vi "Base Run Java Script.vi"(4 "error in":errorcluster, 5 "script args in":string, 6 "script name in":string, 7 "ATS Framework Fields in":T2) -> (0 "error out":errorcluster, 2 "run tool out":T1, 3 "ATS Framework Fields out":T2)   [LabVIEW 2019]
uses:
  <vilib>/Arcadia/Common/Framework/ATS Framework Fields.ctl
  <vilib>/Arcadia/Common/Framework/Run Tool Output.ctl
  <vilib>/Utility/error.llb/whitespace.ctl
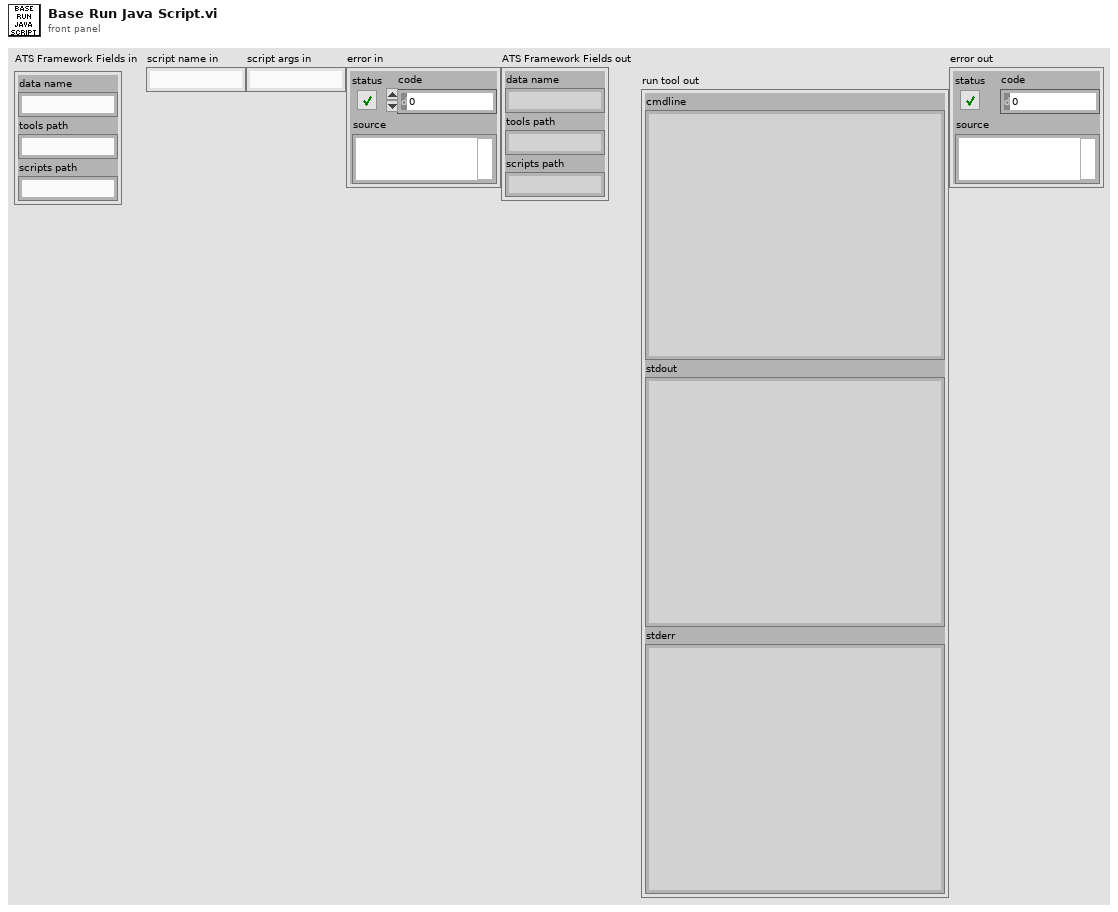
[diagram p1: front panel]
types:
  T1 = typedef "Run Tool Output.ctl" = cluster{"cmdline":string, "stdout":string, "stderr":string}
  T2 = typedef "ATS Framework Fields.ctl" = cluster{"data name":string, "tools path":string, "scripts path":string}
  T3 = typedef "whitespace.ctl" = u16
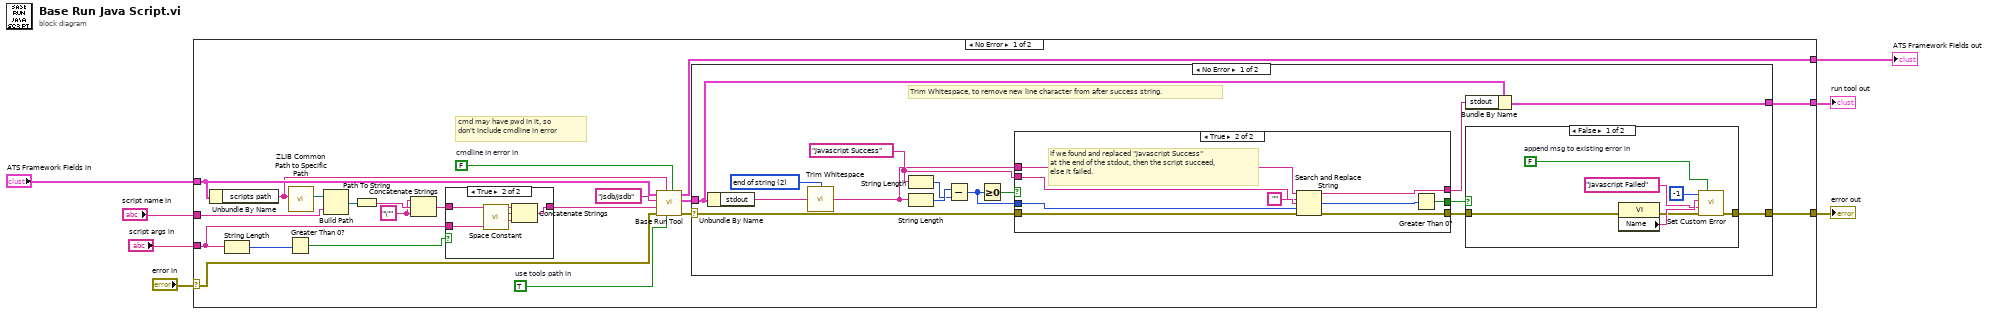
[diagram p0: block diagram]
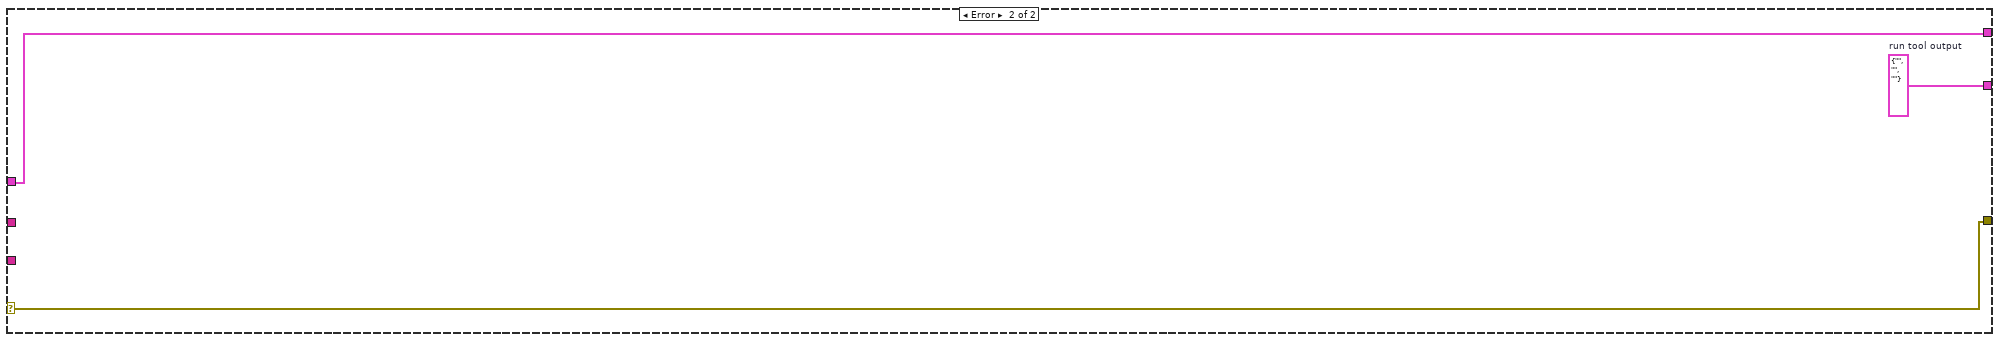
[diagram p6: hidden frame]
diagram:
  n1 = case shown="No Error" "error in" {
    selector: "error in" -> [w20 w73]
    tunnel: [w23 w73] -> w7
    tunnel: "script args in" -> [w14 _]
    tunnel: "ATS Framework Fields in" -> [w22 w72]
    tunnel: "script name in" -> [w24 _]
    tunnel: [w21 w72] -> w2
    tunnel: [w17 w71] -> w1
    frame No Error {
      w8 = FALSE  # cmdline in error in
      w10 = TRUE  # use tools path in
      w25 = "\"" ("string")
      # "cmd may have pwd in it, so\ndon't include cmdline in error"
      n2 = Unbundle By Name(w22) -> ("scripts path"=w9:string)
      n3 = String Length(string=w14) -> (length=w16:i32)
      n4 = Greater Than 0?(x=w16) -> (x > 0?=w15:bool)
      n5 = call <vilib>:"ZLIB Common Path to Specific Path.vi"("common path"=w9) -> ("specific path"=w26:path)  [unwired: 10 in]
      n6 = Build Path(base path=w26, name or relative path=w24) -> (appended path=w28:path)
      n7 = Path To String(path=w28) -> (string=w27:string)
      n8 = Concatenate Strings(w25, w27, w25) -> (w13:string)
      n9 = case shown="True" w15 {
        tunnel: w14 -> [_ w33]
        tunnel: w13 -> [w29 w31]
        tunnel: [w29 w30] -> w12
        frame False {
        }
        frame True {
          n10 = call <vilib>:"Space Constant.vi"() -> ("String"=w32:string)
          n11 = Concatenate Strings(w31, w32, w33) -> (w30:string)
        }
      }
      n12 = call <vilib>:"Base Run Tool.vi"("cmdline in error in"=w8, "use tools path in"=w10, "working directory in"=w9, "error in"=w20, "tool args in"=w12, "tool path in"="jsdb/jsdb" ("command line"), "ATS Framework Fields in"=w22) -> ("error out"=w11:errorcluster, "run tool output"=w18:T1, "ATS Framework Fields out"=w21:T2)  [unwired: 1 in]
      n13 = case shown="No Error" w11 {
        selector: w11 -> [w34 w69]
        tunnel: [w36 w69] -> w23
        tunnel: w18 -> [w40 w70]
        tunnel: [w39 w70] -> w17
        frame No Error {
          w42 = T3 2 items=["both", "start of string", "end of string"] ("location (both)")
          w48 = "Javascript Success" ("search string/char (-)")
          # "Trim Whitespace, to remove new line character from after success string."
          n14 = Unbundle By Name(w40) -> ("stdout"=w41:string)
          n15 = call <vilib>:"Trim Whitespace.vi"("string"=w41, "location (both)"=w42) -> ("trimmed string"=w43:string)
          n16 = String Length(string=w48) -> (length=w46:i32)
          n17 = String Length(string=w43) -> (length=w47:i32)
          n18 = Subtract(x=w47, y=w46) -> (x-y=w45:i32)
          n19 = Greater Or Equal To 0?(x=w45) -> (x >= 0?=w44:bool)
          n20 = case shown="True" w44 {
            selector: w44 -> [w58 _]
            tunnel: w34 -> [w59 w67]
            tunnel: [w59 w65] -> w37
            tunnel: [w58 w64] -> w35
            tunnel: w48 -> [_ w63]
            tunnel: w43 -> [w57 w62]
            tunnel: w45 -> [_ w61]
            tunnel: [w57 w60] -> w38
            frame False {
            }
            frame True {
              # "If we found and replaced \"Javascript Success\"\nat the end of the stdout, then the script succeed,\nelse it failed."
              n21 = Search and Replace String(input string=w62, search string=w63, replace string="" ("replace string (\"\")"), offset=w61, error in=w67) -> (result string=w60:string, number of replacements=w66:i32, error out=w65:errorcluster)  [unwired: 3 in, 1 out]
              n22 = Greater Than 0?(x=w66) -> (x > 0?=w64:bool)
            }
          }
          n23 = Bundle By Name(cluster=w40, "stdout"=w38) -> (w39:T1)
          n24 = case shown="False" w35 {
            tunnel: w37 -> [w52 w56]
            tunnel: [w55 w56] -> w36
            frame False {
              w50 = FALSE  # append msg to existing error in
              n25 = property class="VI"(error in=w52) -> (error out=w51:errorcluster, "Name"=w53:string)  [unwired: 1 in, 1 out]
              n26 = call <vilib>:"Set Custom Error.vi"("append msg to existing error in"=w50, "error in"=w51, "message in"="Javascript Failed", "source in"=w53, "code in"=-1) -> ("error out"=w55:errorcluster)  [unwired: 6 in]
            }
            frame True {
            }
          }
        }
        frame Error {
        }
      }
    }
    frame Error {
      w71 = T1 {"cmdline"="", "stdout"="", "stderr"=""}  # run tool output
    }
  }
  "error out" <- w7
  "ATS Framework Fields out" <- w2
  "run tool out" <- w1
